vi "Format Path and Filename.vi"(8 "error in":errorcluster, 11 "Data in":refnum<class "LV-Data.lvclass">) -> (0 "error out":errorcluster, 3 "Data out":refnum<class "LV-Data.lvclass">)   [LabVIEW 2019, in "LV-Data.lvclass"]
uses:
  LV-Data.lvclass
  LV-Data.lvclass/LV-Data.ctl
  Typedefs/Operation--enum.ctl
panel:
  out "path in":path
  out "formatted path":path
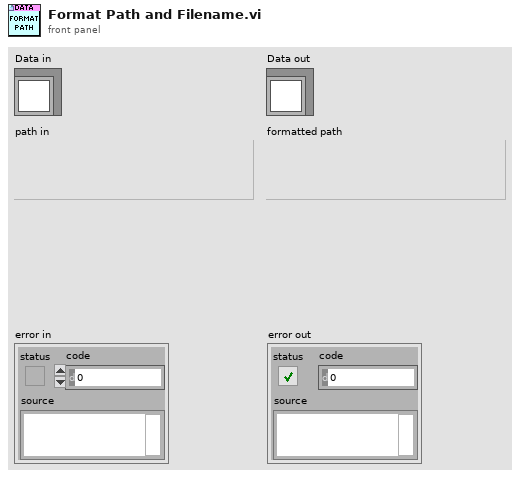
[diagram p1: front panel]
types:
  T1 = typedef "LV-Data.lvclass/Operation--enum.ctl" = enum16{"Read", "Write", "Write + Append"}
  T2 = typedef "LV-Data.lvclass/File Type--enum.ctl" = enum16{"DAT", "ITX", "TDMS", "VI"}
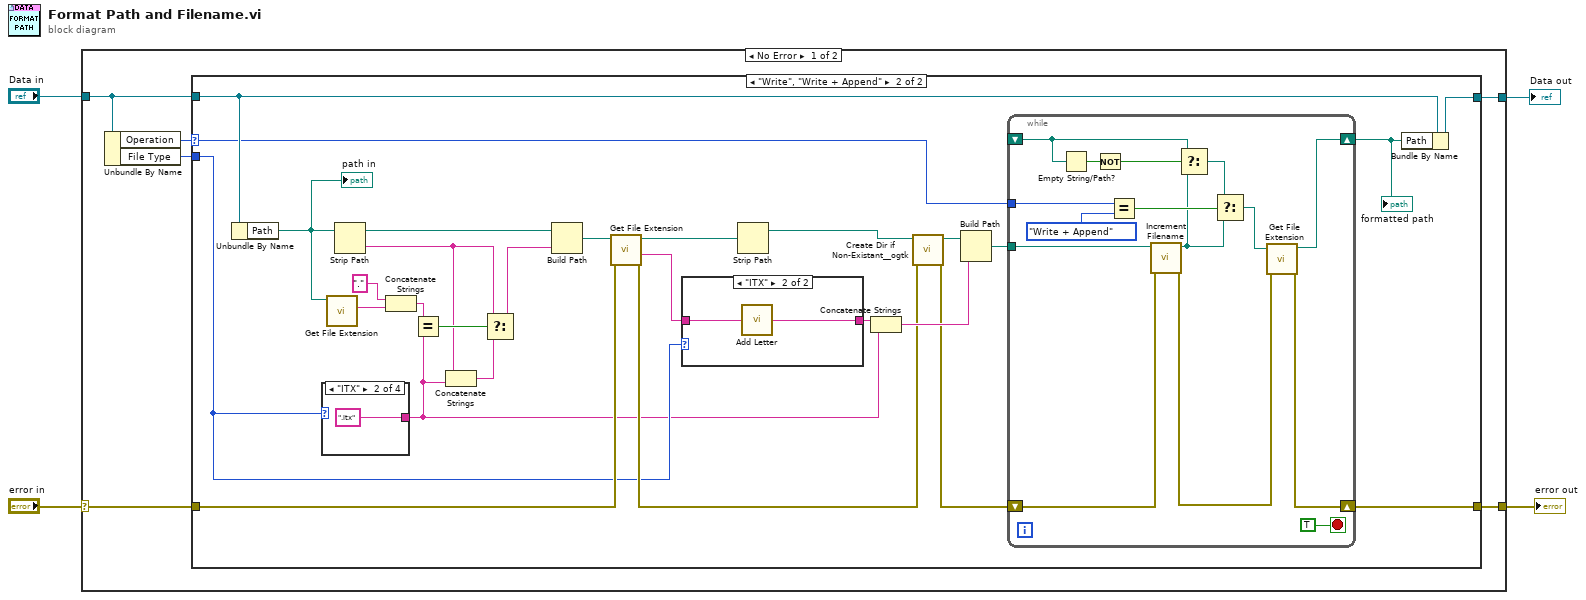
[diagram p0: block diagram]
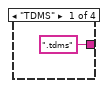
[diagram p4: hidden frame]
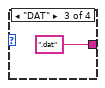
[diagram p5: hidden frame]
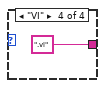
[diagram p6: hidden frame]
diagram:
  n1 = case shown="No Error" "error in" {
    selector: "error in" -> [w9 w63]
    tunnel: [w10 w63] -> w4
    tunnel: "Data in" -> [w7 w62]
    tunnel: [w8 w62] -> w1
    frame No Error {
      n2 = Unbundle By Name(w7) -> ("Operation"=w6:T1, "File Type"=w5:T2)
      n3 = case shown="\"Write\", \"Write + Append\"" w6 {
        selector: w6 -> [_ w26]
        tunnel: [w11 w37] -> w10
        tunnel: w9 -> [w11 w23]
        tunnel: [w12 w29] -> w8
        tunnel: w7 -> [w12 w28]
        tunnel: w5 -> [_ w22]
        frame "Read", Default {
        }
        frame "Write", "Write + Append" {
          n4 = Unbundle By Name(w28) -> ("Path"=w13:path)
          "path in" <- w13
          n5 = case shown="\"ITX\"" w22 {
            tunnel: [".tdms" ("string") ".itx" ("string") ".dat" ("string") ".vi" ("string")] -> w15
            frame "TDMS" {
            }
            frame "ITX" {
            }
            frame "DAT" {
            }
            frame "VI" {
            }
          }
          n6 = call <vilib>:"Get File Extension.vi"("file"=w13) -> ("lowercase file extension"=w20:string)  [unwired: 6 in, 4 out]
          n7 = Strip Path(path=w13) -> (stripped path=w25:path, name=w17:string)
          n8 = Concatenate Strings("." ("string"), w20) -> (w19:string)
          n9 = Equal?(x=w19, y=w15) -> (x = y?=w18:bool)
          n10 = Concatenate Strings(w17, w15) -> (w14:string)
          n11 = Select(t=w17, s=w18, f=w14) -> (s? t:f=w16:string)
          n12 = Build Path(base path=w25, name or relative path=w16) -> (appended path=w24:path)
          n13 = call <vilib>:"Get File Extension.vi"("error in (no error)"=w23, "file"=w24) -> ("error out"=w31:errorcluster, "filename without extension"=w32:string, "dup file"=w34:path)  [unwired: 7 out]
          n14 = case shown="\"ITX\"" w22 {
            tunnel: [w40 w42] -> w38
            tunnel: w32 -> [w40 w41]
            frame Default {
            }
            frame "ITX" {
              n15 = call "Add Letter.vi"("string"=w41) -> ("result string"=w42:string)
            }
          }
          n16 = Strip Path(path=w34) -> (stripped path=w33:path)  [unwired: 1 out]
          n17 = Concatenate Strings(w38, w15) -> (w39:string)
          n18 = call <userlib>:"Create Dir if Non-Existant__ogtk.vi"("error in (no error)"=w31, "Directory Path"=w33) -> ("error out"=w36:errorcluster, "dup Directory Path"=w30:path)  [unwired: 7 in, 1 out]
          n19 = Build Path(base path=w30, name or relative path=w39) -> (appended path=w35:path)
          n20 = while {
            tunnel: w26 -> [w47]
            tunnel: w35 -> [w45]
            shift-right: [w51] -> w27
            shift-left: _ -> [w54]
            shift-right: [w53] -> w37
            shift-left: w36 -> [w50]
            stop <- TRUE stop-if-true
            n21 = Empty String/Path?(string/path=w54) -> (empty?=w56:bool)
            n22 = Not(x=w56) -> (.not. x?=w55:bool)
            n23 = Equal?(x=w47, y=Operation--enum."Write + Append" ("Operation")) -> (x = y?=w46:bool)
            n24 = call <userlib>:"Increment Filename.vi"("error in (no error)"=w50, "Path"=w45) -> ("error out"=w49:errorcluster, "Modified Path"=w44:path)  [unwired: 8 in]
            n25 = Select(t=w54, s=w55, f=w44) -> (s? t:f=w43:path)
            n26 = Select(t=w43, s=w46, f=w44) -> (s? t:f=w52:path)
            n27 = call <vilib>:"Get File Extension.vi"("error in (no error)"=w49, "file"=w52) -> ("error out"=w53:errorcluster, "dup file"=w51:path)  [unwired: 8 out]
          }
          "formatted path" <- w27
          n28 = Bundle By Name(cluster=w28, "Path"=w27) -> (w29:refnum<class "LV-Data.lvclass">)
        }
      }
    }
    frame Error {
    }
  }
  "error out" <- w4
  "Data out" <- w1
